vi "Si Material Properties.vi"(6 "NS Base Area":dbl, 9 "m-nm Si":dbl, 10 "Silicon Thickness in":dbl, 11 "Energy (Heat; I^2R)":dbl) -> (0 "Volume Si":dbl, 1 "Silicon Density":dbl, 2 "Delta Temp Change Si":dbl, 3 "Silicon Specfic Heat Capacity":dbl, 4 "Silicon Thickness out":dbl, 5 "Mass Si":dbl)   [LabVIEW 2020]
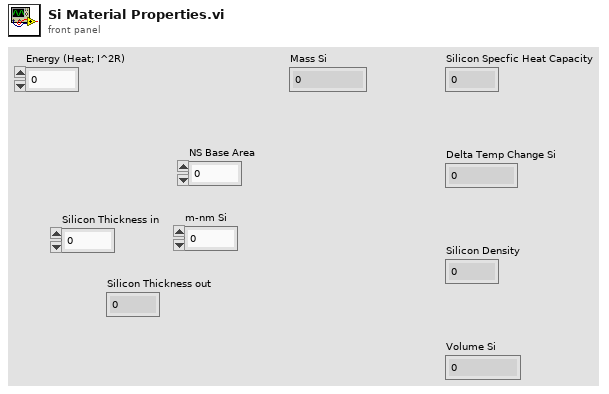
[diagram p1: front panel]
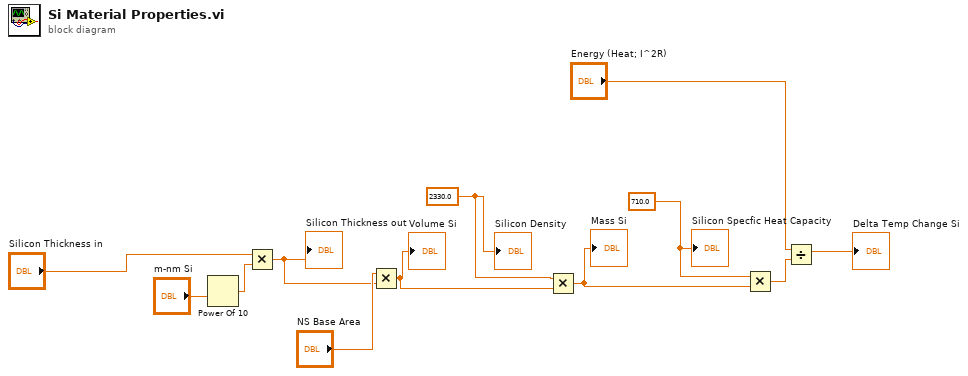
[diagram p0: block diagram]
diagram:
  w9 = 710.0 ("Silicon Specfic Heat Capacity")
  w6 = 2330.0 ("Silicon Density")
  n1 = Power Of 10(x="m-nm Si") -> (10^x=w1:dbl)
  n2 = Multiply(x="Silicon Thickness in", y=w1) -> (x*y=w4:dbl)
  "Silicon Thickness out" <- w4
  n3 = Multiply(x="NS Base Area", y=w4) -> (x*y=w5:dbl)
  "Volume Si" <- w5
  n4 = Multiply(x=w6, y=w5) -> (x*y=w10:dbl)
  "Mass Si" <- w10
  n5 = Multiply(x=w9, y=w10) -> (x*y=w7:dbl)
  n6 = Divide(x="Energy (Heat; I^2R)", y=w7) -> (x/y=→"Delta Temp Change Si":dbl)
  "Silicon Density" <- w6
  "Silicon Specfic Heat Capacity" <- w9
